vi "Verify end axis (SubVI).vi"(5 "error in":errorcluster, 8 "VISA Refnum in":refnum<visa-resource-name>) -> (0 "error out":errorcluster, 1 "time, sec":i32, 2 "progress, %":i32, 3 "VISA resource name out":refnum<visa-resource-name>)   [LabVIEW 2018]
uses:
  GlobalStop.vi
panel:
  out "err":errorcluster
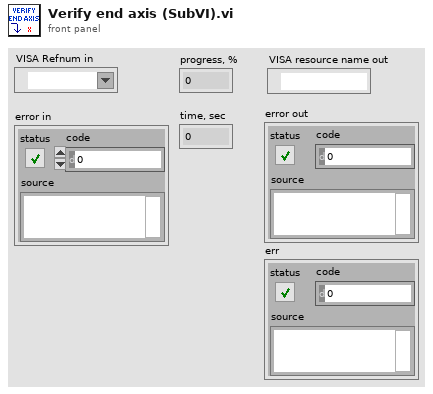
[diagram p1: front panel]
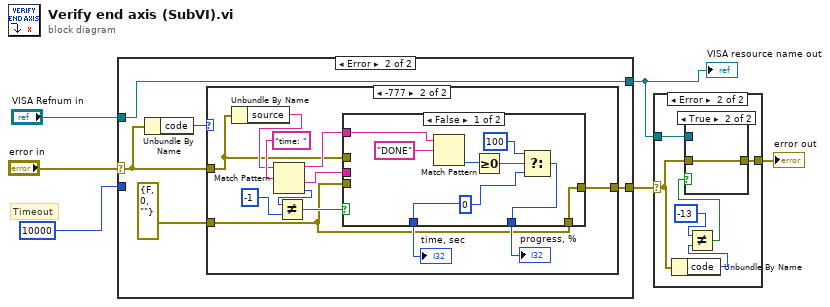
[diagram p0: block diagram]
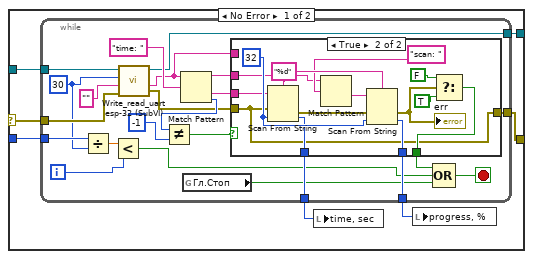
[diagram p4: hidden frame]
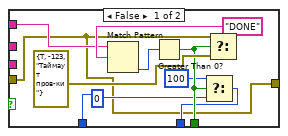
[diagram p5: hidden frame]
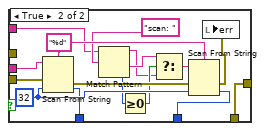
[diagram p7: hidden frame]
diagram:
  # "Timeout"
  n1 = case shown="Error" "error in" {
    selector: "error in" -> [w12 w61]
    tunnel: "VISA Refnum in" -> [w13 w64]
    tunnel: 10000 -> [w11 _]
    tunnel: [w10 w64] -> w2
    tunnel: [w9 w62] -> w3
    frame No Error {
      n2 = while {
        tunnel: w13 -> [w36]
        tunnel: w12 -> [w34]
        tunnel: w11 -> [w33]
        tunnel: [w21] -> w10
        tunnel: [w22] -> w9
        tunnel: [w20] -> w8
        tunnel: [w19] -> w7
        i -> [w30]
        stop <- w29 stop-if-true
        w32 = u32 30 ("milliseconds to wait")
        n3 = Divide(x=w33, y=w32) -> (x/y=w31:dbl)
        n4 = Less?(x=w31, y=w30) -> (x < y?=w15:bool)
        n5 = call "Write_read_uart esp-32 (SubVI).vi"("error in (no error)"=w34, "write buffer"="", "milliseconds to wait"=w32, "VISA Refnum in"=w36) -> ("error out 4"=w25:errorcluster, "read buffer"=w16:string, "VISA resource name out"=w21:refnum<visa-resource-name>)  [unwired: 1 out]
        n6 = Match Pattern(string=w16, regular expression="time: ") -> (before substring=w24:string, after substring=w23:string, offset past match=w26:i32)  [unwired: 1 in, 1 out]
        n7 = Not Equal?(x=w26, y=-1 ("offset past match")) -> (x != y?=w18:bool)
        n8 = global read "GlobalStop.vi" "Гл.Стоп"() -> (w14:bool)
        n9 = case shown="True" w18 {
          tunnel: w25 -> [w37 w46]
          tunnel: w24 -> [_ w51]
          tunnel: w23 -> [_ w52]
          tunnel: [w37 w46] -> w22
          tunnel: [w40 w56] -> w20
          tunnel: [w39 w55] -> w19
          tunnel: [w41 w47] -> w17
          tunnel: w16 -> [w43 _]
          frame False {
            w40 = 0 ("default value 1")
            n10 = Match Pattern(string=w43, regular expression="DONE") -> (offset past match=w44:i32)  [unwired: 1 in, 3 out]
            n11 = Greater Than 0?(x=w44) -> (x > 0?=w41:bool)
            n12 = Select(t=100, s=w41, f=w40) -> (s? t:f=w39:i32)
            n13 = Select(t=w37, s=w41, f=errorcluster {"status"=TRUE, "code"=-123, "source"="Таймаут пров-ки"} ("error constant")) -> ()  [unwired: 1 out]
          }
          frame True {
            w57 = 32 ("default value 1")
            w59 = "%d" ("format string")
            n14 = Scan From String(format string=w59, input string=w52, error in=w46, default 1=w57) -> (error out=w58:errorcluster, output 1=w56:i32)  [unwired: 1 in, 2 out]
            n15 = Match Pattern(string=w51, regular expression="scan: ") -> (after substring=w53:string)  [unwired: 1 in, 3 out]
            n16 = Scan From String(format string=w59, input string=w53, error in=w58, default 1=w57) -> (error out=w50:errorcluster, output 1=w55:i32)  [unwired: 1 in, 2 out]
            "err" <- w50
            n17 = Select(t=FALSE, s=w50, f=TRUE) -> (s? t:f=w47:bool)
          }
        }
        n18 = Compound Arithmetic op=OR(w17, w15, w14) -> (w29:bool)
      }
      n19 = local write "time, sec"(w8) -> ()
      n20 = local write "progress, %"(w7) -> ()
    }
    frame Error {
      n21 = Unbundle By Name(w61) -> ("code"=w60:i32)
      n22 = case shown="-777" w60 {
        tunnel: w61 -> [w65 w70]
        tunnel: errorcluster {"status"=FALSE, "code"=0, "source"=""} ("error constant") -> [_ w66]
        tunnel: [w65 w69] -> w62
        frame 0, Default {
        }
        frame -777 {
          n23 = Unbundle By Name(w70) -> ("source"=w71:string)
          n24 = Match Pattern(string=w71, regular expression="time: ") -> (before substring=w72:string, after substring=w73:string, offset past match=w75:i32)  [unwired: 1 in, 1 out]
          n25 = Not Equal?(x=w75, y=-1 ("offset past match")) -> (x != y?=w74:bool)
          n26 = case shown="False" w74 {
            tunnel: w66 -> [_ w101]
            tunnel: w72 -> [w85 w94]
            tunnel: w73 -> [_ w95]
            tunnel: [w81 w97] -> w68
            tunnel: [w80 w93] -> w67
            tunnel: w70 -> [_ _]
            tunnel: [w78 w87] -> w69
            tunnel: w66 -> [w78 w87]
            frame False {
              w81 = 0 ("default value 1")
              n27 = Match Pattern(string=w85, regular expression="DONE") -> (offset past match=w84:i32)  [unwired: 1 in, 3 out]
              n28 = Greater Or Equal To 0?(x=w84) -> (x >= 0?=w82:bool)
              n29 = Select(t=100, s=w82, f=w81) -> (s? t:f=w80:i32)
            }
            frame True {
              w98 = 32 ("default value 1")
              w100 = "%d" ("format string")
              n30 = Scan From String(format string=w100, input string=w95, error in=w101, default 1=w98) -> (error out=w99:errorcluster, output 1=w97:i32)  [unwired: 1 in, 2 out]
              n31 = Match Pattern(string=w94, regular expression="scan: ") -> (before substring=w89:string, after substring=w90:string, offset past match=w92:i32)  [unwired: 1 in, 1 out]
              n32 = Greater Or Equal To 0?(x=w92) -> (x >= 0?=w91:bool)
              n33 = Select(t=w90, s=w91, f=w89) -> (s? t:f=w88:string)
              n34 = Scan From String(format string=w100, input string=w88, error in=w99, default 1=w98) -> (error out=w86:errorcluster, output 1=w93:i32)  [unwired: 1 in, 2 out]
              n35 = local write "err"(w86) -> ()
            }
          }
          "time, sec" <- w68
          "progress, %" <- w67
        }
      }
    }
  }
  "VISA resource name out" <- w2
  n36 = case shown="Error" w3 {
    selector: w3 -> [w102 w103]
    tunnel: w2 -> [_ w108]
    tunnel: [w102 w107] -> w1
    frame No Error {
    }
    frame Error {
      n37 = Unbundle By Name(w103) -> ("code"=w106:i32)
      n38 = Not Equal?(x=-13, y=w106) -> (x != y?=w104:bool)
      n39 = case shown="True" w104 {
        tunnel: w108 -> [_ _]
        tunnel: [w109 w110] -> w107
        tunnel: w103 -> [w109 w110]
        frame False {
        }
        frame True {
        }
      }
    }
  }
  "error out" <- w1
